vi "DecorateTable.vi"(6 "Elapsed Time":dbl, 7 "Current Temperature":dbl, 8 "error in (no error)":errorcluster, 9 "Current Program":dbl, 10 "Tbl Refnum":refnum<vi>, 11 "RampTable":string[][](array[string])) -> (0 "error out":errorcluster)   [LabVIEW 2013]
doc: "Use this template to build a VI to use as a subVI."
uses:
  <vilib>/Utility/miscctls.llb/LVRowAndColumnTypeDef.ctl
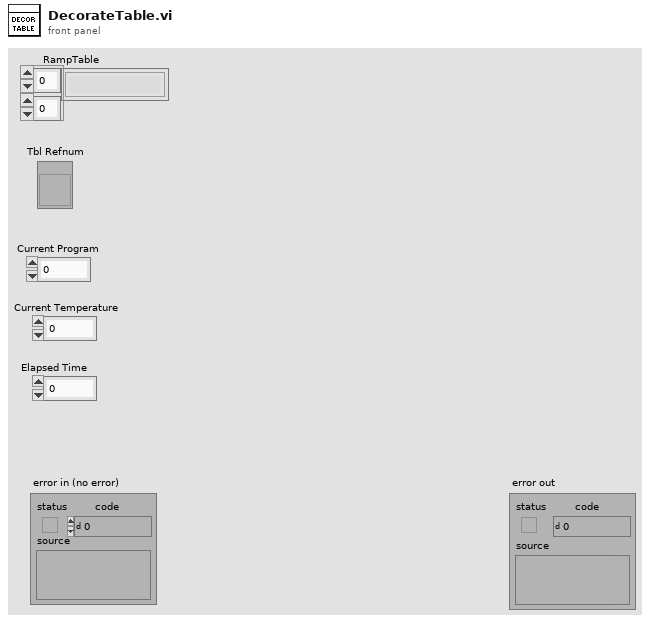
[diagram p1: front panel]
types:
  T1 = typedef "LVRowAndColumnTypeDef.ctl" = cluster{"Row":i32, "Column":i32}
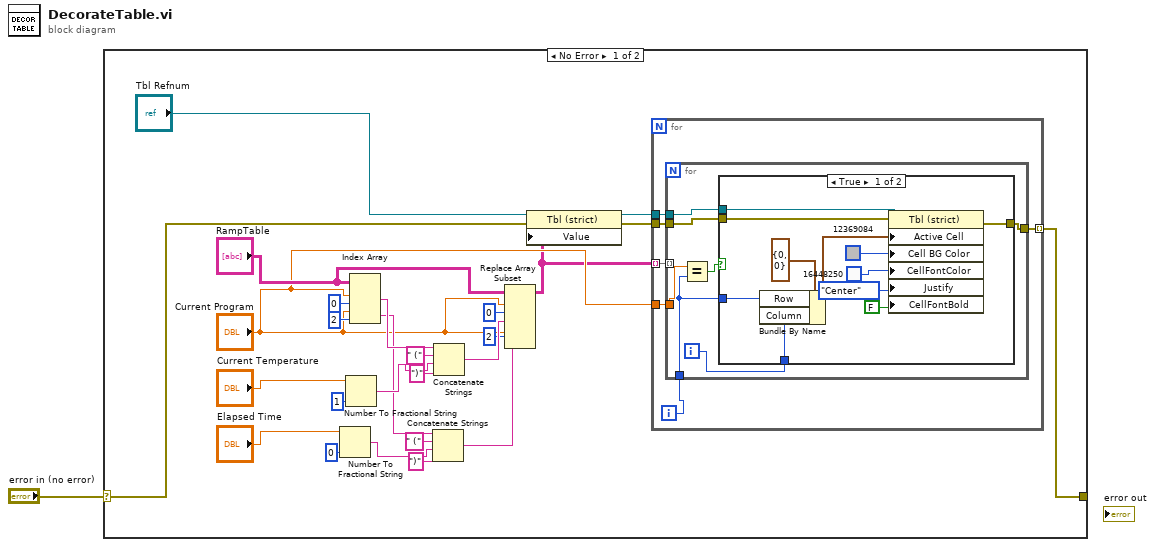
[diagram p0: block diagram]
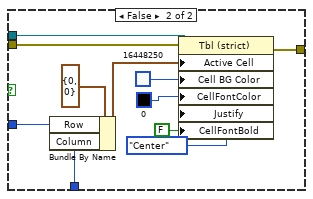
[diagram p2: hidden frame]
diagram:
  n1 = case shown="No Error" "error in (no error)" {
    selector: "error in (no error)" -> [w5 _]
    tunnel: [w4 _] -> _
    frame No Error {
      n2 = Number To Fractional String(number="Elapsed Time", precision (6)=i16 0) -> (F-format string=w11:string)  [unwired: 2 in]
      n3 = Number To Fractional String(number="Current Temperature", precision (6)=i16 1) -> (F-format string=w20:string)  [unwired: 2 in]
      n4 = Index Array(array="RampTable", index (row) #1="Current Program", index (col) #1=0 ("disabled index (col)"), index (row) #2="Current Program", index (col) #2=2 ("disabled index (col)")) -> (element #1=w24:string, element #2=w13:string)
      n5 = Concatenate Strings(w13, " (" ("string"), w11, ")" ("string")) -> (w8:string)
      n6 = Concatenate Strings(w24, " (" ("string"), w20, ")" ("string")) -> (w16:string)
      n7 = Replace Array Subset(array="RampTable", new element #1=w16, index (row) #1="Current Program", index (col) #1=0 ("disabled index (col)"), new element #2=w8, index (row) #2="Current Program", index (col) #2=2 ("disabled index (col)")) -> (w2:string[][])
      n8 = property class="Tbl (strict)"(reference="Tbl Refnum", error in=w5, "Value"=w2) -> (reference out=w7:refnum<vi>, error out=w6:errorcluster)
      n9 = for {
        tunnel: w7 -> [w33]
        tunnel: w6 -> [w32]
        tunnel: [w31] -> w4 mode=indexing
        tunnel: "Current Program" -> [w30]
        tunnel: w2 -> [w29] mode=indexing
        i -> [w28]
        n10 = for {
          tunnel: w33 -> [w40]
          tunnel: w32 -> [w39]
          tunnel: [w38] -> w31
          tunnel: w30 -> [w36]
          tunnel: w29 -> [_] mode=indexing
          tunnel: w28 -> [w34]
          i -> [w37]
          n11 = Equal?(x=w36, y=w34) -> (x = y?=w35:bool)
          n12 = case shown="True" w35 {
            tunnel: w40 -> [w51 w62]
            tunnel: w39 -> [w50 w61]
            tunnel: [w49 w60] -> w38
            tunnel: w37 -> [w47 w58]
            tunnel: w34 -> [w43 w54]
            frame True {
              n13 = Bundle By Name(cluster=T1 {"Row"=0, "Column"=0} ("Active Cell:Active Cell"), "Row"=w43, "Column"=w47) -> (w46:T1)
              n14 = property class="Tbl (strict)"(reference=w51, error in=w50, "Active Cell"=w46, "Cell BG Color"=u32 12369084 ("Color"), "CellFontColor"=u32 16448250 ("Color"), "Justify"=enum16{"Left", "Center", "Right"}."Center" ("Active Cell:Cell Justification"), "CellFontBold"=FALSE ("Active Cell:Cell Font:Bold")) -> (error out=w49:errorcluster)  [unwired: 1 out]
            }
            frame False {
              n15 = Bundle By Name(cluster=T1 {"Row"=0, "Column"=0} ("Active Cell:Active Cell"), "Row"=w54, "Column"=w58) -> (w57:T1)
              n16 = property class="Tbl (strict)"(reference=w62, error in=w61, "Active Cell"=w57, "Cell BG Color"=u32 16448250 ("Color"), "CellFontColor"=u32 0 ("Color"), "Justify"=enum16{"Left", "Center", "Right"}."Center" ("Active Cell:Cell Justification"), "CellFontBold"=FALSE ("Active Cell:Cell Font:Bold")) -> (error out=w60:errorcluster)  [unwired: 1 out]
            }
          }
        }
      }
    }
    frame Error {
    }
  }
